vi "TEST - Empty Array.vi"(8 "error in (no error)":errorcluster) -> (0 "error out":errorcluster, 2 "Pass?":bool=TRUE)   [LabVIEW 2009]
doc: "This VI template can be used for the functional testing of VIs; this implementation includes handling for the testing of polymorphic VIs, and the polymorphic elements should be removed if not needed.\n\nCoded by Douglas A. Femec, January 24, 2006.\n\nCopyright (c) 2005-2006 MKS Instruments, Inc.\nAll rights reserved."
uses:
  TEST - Empty Array - Inputs.ctl
  Polymorphizer+ Data Type.ctl
  TEST - Empty Array - Outputs.ctl
  source/library/Empty Array/Empty 1D Array (EXT).vi
  source/library/Empty Array/Empty 2D Array (EXT).vi
  source/library/Empty Array/Empty 1D Array (I64).vi
  source/library/Empty Array/Empty 2D Array (I64).vi
  source/library/Empty Array/Empty 1D Array (U64).vi
  source/library/Empty Array/Empty 2D Array (U64).vi
  source/library/Empty Array/Empty 1D Array (DBL).vi
  source/library/Empty Array/Empty 2D Array (DBL).vi
  source/library/Empty Array/Empty 1D Array (SGL).vi
  source/library/Empty Array/Empty 2D Array (SGL).vi
  source/library/Empty Array/Empty 1D Array (I32).vi
  source/library/Empty Array/Empty 2D Array (I32).vi
  source/library/Empty Array/Empty 1D Array (I16).vi
  source/library/Empty Array/Empty 2D Array (I16).vi
  source/library/Empty Array/Empty 1D Array (I8).vi
  source/library/Empty Array/Empty 2D Array (I8).vi
  source/library/Empty Array/Empty 1D Array (LVObject).vi
  source/library/Empty Array/Empty 2D Array (LVObject).vi
  source/library/Empty Array/Empty 1D Array (U32).vi
  source/library/Empty Array/Empty 2D Array (U32).vi
  source/library/Empty Array/Empty 1D Array (U16).vi
  source/library/Empty Array/Empty 2D Array (U16).vi
  source/library/Empty Array/Empty 1D Array (U8).vi
  source/library/Empty Array/Empty 2D Array (U8).vi
  source/library/Empty Array/Empty 1D Array (CXT).vi
  source/library/Empty Array/Empty 2D Array (CXT).vi
  source/library/Empty Array/Empty 1D Array (CDB).vi
  source/library/Empty Array/Empty 2D Array (CDB).vi
  source/library/Empty Array/Empty 1D Array (CSG).vi
  source/library/Empty Array/Empty 2D Array (CSG).vi
  source/library/Empty Array/Empty 1D Array (Boolean).vi
  source/library/Empty Array/Empty 2D Array (Boolean).vi
  source/library/Empty Array/Empty 1D Array (String).vi
  source/library/Empty Array/Empty 2D Array (String).vi
  source/library/Empty Array/Empty 1D Array (Path).vi
  source/library/Empty Array/Empty 2D Array (Path).vi
  source/library/Empty Array/Empty Array (Variant).vi
  source/library/Empty Array/Empty 1D Array (Variant).vi
  source/library/Empty Array/Empty 2D Array (Variant).vi
  TestClass/TestClass.lvclass
panel:
  out "Generated Outputs":T1[][](array[typedef])
  in  "Expected Outputs":T1[](array[typedef])=[{"Description"="Expect true", "1D Empty?"=TRUE, "2D Empty?"=TRUE}, {"Description"="Expect false", "1D Empty?"=FALSE, "2D Empty?"=FALSE}, {"Description"="Expect false", "1D Empty?"=FALSE, "2D Empty?"=FALSE}]
  in  "Inputs":T2[](array[typedef])=[{"Description"="Empty arrays", "Data Types to Test"=[enum."EXT", enum."DBL", enum."SGL", enum."I32", enum."I16", enum."I8", enum."U32", enum."U16", enum."U8", enum."CXT", enum."CDB", enum."CSG", enum."Boolean", enum."String", enum."Path", enum."Variant", enum."I64", enum."U64", enum."LabVIEW Object"], "1D Array"=[], "2D Array"=[]}, {"Description"="One-element arrays", "Data Types to Test"=[enum."EXT", enum."DBL", enum."SGL", enum."I32", enum."I16", enum."I8", enum."U32", enum."U16", enum."U8", enum."CXT", enum."CDB", enum."CSG", enum."Boolean", enum."String", enum."Path", enum."Variant", enum."I64", enum."U64", enum."LabVIEW Object"], "1D Array"=[0.0], "2D Array"=[[0.0]]}, {"Description"="Multi-element arrays", "Data Types to Test"=[enum."EXT", enum."DBL", enum."SGL", enum."I32", enum."I16", enum."I8", enum."U32", enum."U16", enum."U8", enum."CXT", enum."CDB", enum."CSG", enum."Boolean", enum."String", enum."Path", enum."Variant", enum."I64", enum."U64", enum."LabVIEW Object"], "1D Array"=[1.0, 0.0, 1.0, 1.0], "2D Array"=[[0.0, 0.0], [1.0, 0.0], [1.0, 1.0]]}] {"1D Array" format="%.2f"; "2D Array" format="%.2f"}
  # "Copyright (c) 2005-2006 MKS Instruments, Inc.\nAll rights reserved."
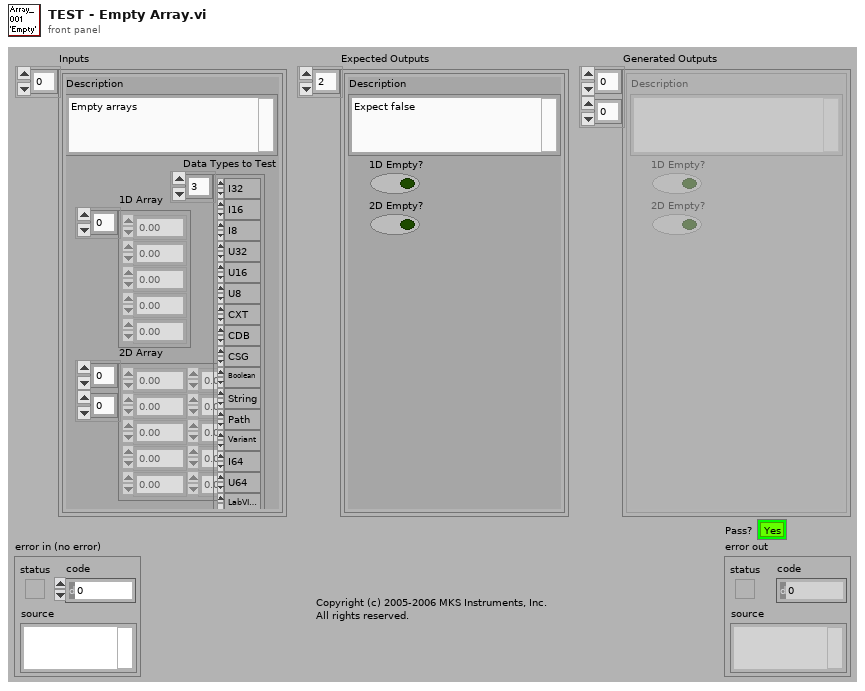
[diagram p1: front panel]
types:
  T1 = typedef "TEST - Empty Array - Outputs.ctl" = cluster{"Description":string, "1D Empty?":bool, "2D Empty?":bool}
  T2 = typedef "TEST - Empty Array - Inputs.ctl" = cluster{"Description":string, "Data Types to Test":T3[], "1D Array":sgl[], "2D Array":sgl[][]}
  T3 = typedef "Polymorphizer+ Data Type.ctl" = enum16{"EXT", "DBL", "SGL", "I32", "I16", "I8", "U32", "U16", "U8", "CXT", "CDB", "CSG", "Boolean", "String", "Path", "Variant", "CTL-REF", "GEN-REF", "GObj-REF", "VI-REF", "ENUM", "ERR", "FILE-REF", "MENU-REF", "MENU-RING", "PICT-RING", "TXT&PICT-RING", "TXT-RING", "I64", "U64", "LabVIEW Object"}
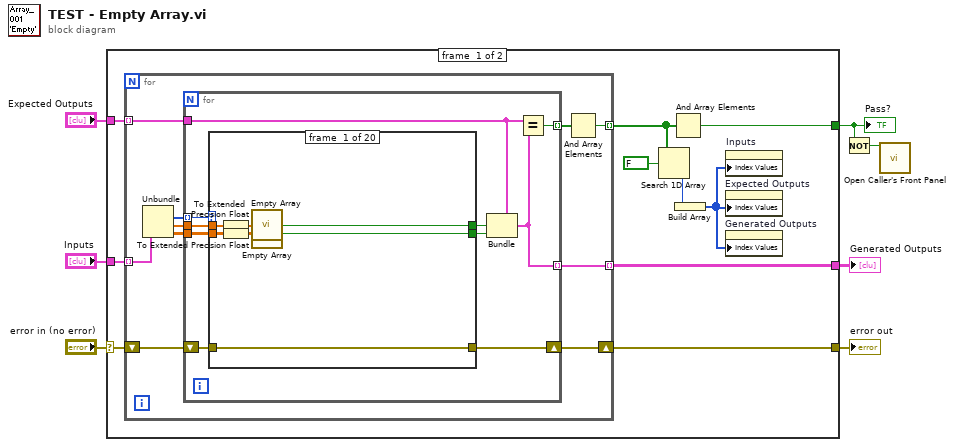
[diagram p0: block diagram]
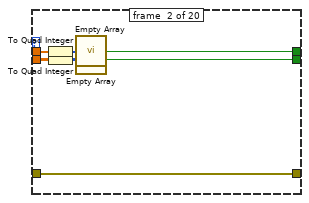
[diagram p2: hidden frame]
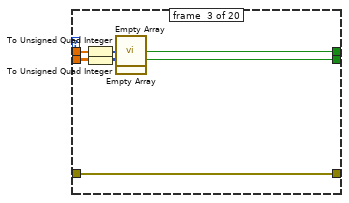
[diagram p3: hidden frame]
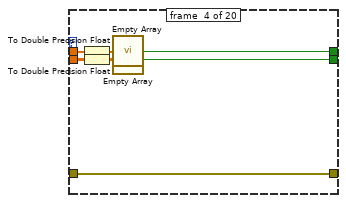
[diagram p4: hidden frame]
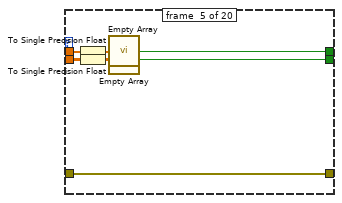
[diagram p5: hidden frame]
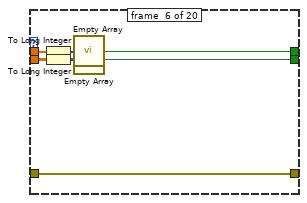
[diagram p6: hidden frame]
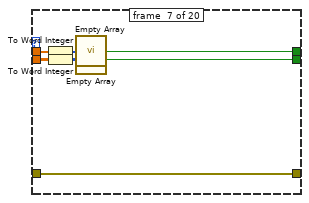
[diagram p7: hidden frame]
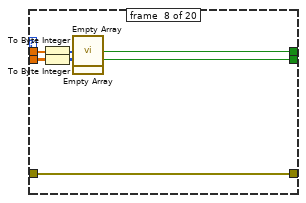
[diagram p8: hidden frame]
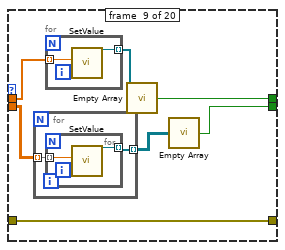
[diagram p9: hidden frame]
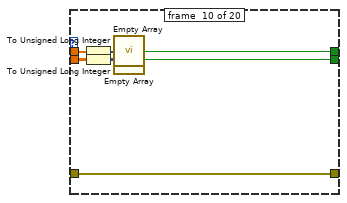
[diagram p10: hidden frame]
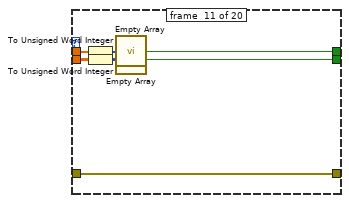
[diagram p11: hidden frame]
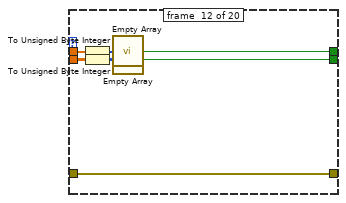
[diagram p12: hidden frame]
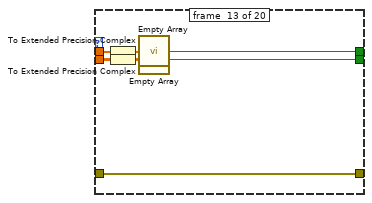
[diagram p13: hidden frame]
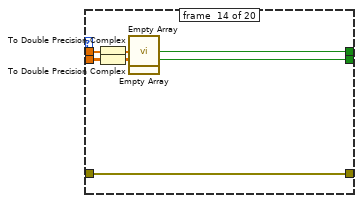
[diagram p14: hidden frame]
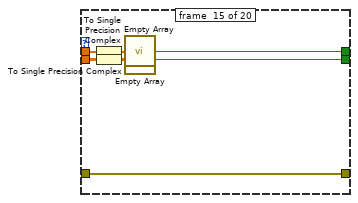
[diagram p15: hidden frame]
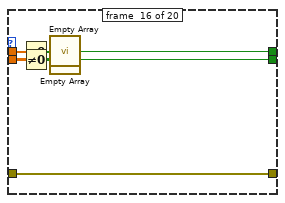
[diagram p16: hidden frame]
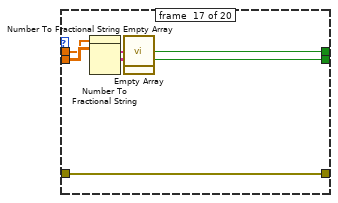
[diagram p17: hidden frame]
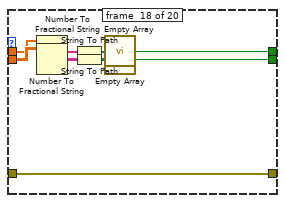
[diagram p18: hidden frame]
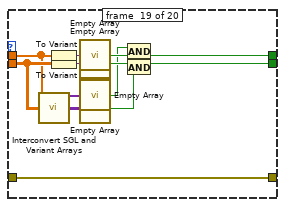
[diagram p19: hidden frame]
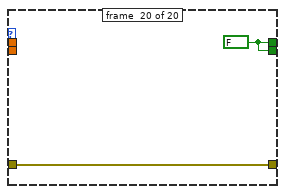
[diagram p20: hidden frame]
diagram:
  n1 = case shown="No Error" "error in (no error)" {
    selector: "error in (no error)" -> [w16 w187]
    tunnel: [w17 w187] -> w6
    tunnel: "Expected Outputs" -> [w14 _]
    tunnel: "Inputs" -> [w15 _]
    tunnel: [w13 _] -> w3
    tunnel: [w12 _] -> w1
    frame #0 {
      n2 = for {
        shift-right: [w22] -> w17
        shift-left: w16 -> [w23]
        tunnel: w15 -> [w24] mode=indexing
        tunnel: w14 -> [w27] mode=indexing
        tunnel: [w26] -> w13 mode=indexing
        tunnel: [w21] -> w11 mode=indexing
        n3 = Unbundle(w24) -> ("Data Types to Test"=w20:T3[], "1D Array"=w19:sgl[], "2D Array"=w18:sgl[][])  [unwired: 1 out]
        n4 = for {
          tunnel: w27 -> [w37]
          tunnel: [w35] -> w26 mode=indexing
          tunnel: [w36] -> w25 mode=indexing
          shift-right: [w30] -> w22
          shift-left: w23 -> [w31]
          tunnel: w20 -> [w32] mode=indexing
          tunnel: w19 -> [w34]
          tunnel: w18 -> [w33]
          n5 = case shown="\"LabVIEW Object\"" w32 {
            tunnel: w34 -> [w43 w50 w57 w64 w71 w78 w85 w92 w97 w112 w119 w126 w133 w140 w147 w154 w159 w168 w173 _]
            tunnel: [w39 w46 w53 w60 w66 w73 w80 w87 w98 w107 w114 w121 w128 w135 w142 w150 w157 w164 w177 w186] -> w29
            tunnel: [w38 w45 w52 w59 w67 w74 w81 w88 w99 w108 w115 w122 w129 w136 w143 w149 w156 w163 w175 w186] -> w28
            tunnel: w33 -> [w44 w51 w58 w65 w72 w79 w86 w93 w94 w113 w120 w127 w134 w141 w148 w155 w161 w170 w179 _]
            tunnel: w31 -> [w40 w47 w54 w61 w68 w75 w82 w89 w100 w109 w116 w123 w130 w137 w144 w151 w158 w165 w184 w185]
            tunnel: [w40 w47 w54 w61 w68 w75 w82 w89 w100 w109 w116 w123 w130 w137 w144 w151 w158 w165 w184 w185] -> w30
            frame #0 {
              n6 = To Extended Precision Float(1:w43) -> (0:w42:ext[])
              n7 = To Extended Precision Float(1:w44) -> (0:w41:ext[][])
              n8 = call-poly "Empty Array.vi"("Array"=w42) -> ("Empty Array?"=w39:bool)  [unwired: 8 in]
              n9 = call-poly "Empty Array.vi"("Array"=w41) -> ("Empty Array?"=w38:bool)  [unwired: 8 in]
            }
            frame #1 {
              n10 = To Quad Integer(1:w50) -> (0:w49:i64[])
              n11 = To Quad Integer(1:w51) -> (0:w48:i64[][])
              n12 = call-poly "Empty Array.vi"("Array"=w49) -> ("Empty Array?"=w46:bool)  [unwired: 8 in]
              n13 = call-poly "Empty Array.vi"("Array"=w48) -> ("Empty Array?"=w45:bool)  [unwired: 8 in]
            }
            frame #2 {
              n14 = To Unsigned Quad Integer(1:w57) -> (0:w56:u64[])
              n15 = To Unsigned Quad Integer(1:w58) -> (0:w55:u64[][])
              n16 = call-poly "Empty Array.vi"("Array"=w56) -> ("Empty Array?"=w53:bool)  [unwired: 8 in]
              n17 = call-poly "Empty Array.vi"("Array"=w55) -> ("Empty Array?"=w52:bool)  [unwired: 8 in]
            }
            frame #3 {
              n18 = To Double Precision Float(number=w64) -> (double precision float=w63:dbl[])
              n19 = To Double Precision Float(number=w65) -> (double precision float=w62:dbl[][])
              n20 = call-poly "Empty Array.vi"("Array"=w63) -> ("Empty Array?"=w60:bool)  [unwired: 8 in]
              n21 = call-poly "Empty Array.vi"("Array"=w62) -> ("Empty Array?"=w59:bool)  [unwired: 8 in]
            }
            frame #4 {
              n22 = To Single Precision Float(number=w71) -> (single precision float=w70:sgl[])
              n23 = To Single Precision Float(number=w72) -> (single precision float=w69:sgl[][])
              n24 = call-poly "Empty Array.vi"("Array"=w70) -> ("Empty Array?"=w66:bool)  [unwired: 8 in]
              n25 = call-poly "Empty Array.vi"("Array"=w69) -> ("Empty Array?"=w67:bool)  [unwired: 8 in]
            }
            frame #5 {
              n26 = To Long Integer(number=w78) -> (32bit integer=w77:i32[])
              n27 = To Long Integer(number=w79) -> (32bit integer=w76:i32[][])
              n28 = call-poly "Empty Array.vi"("Array"=w77) -> ("Empty Array?"=w73:bool)  [unwired: 8 in]
              n29 = call-poly "Empty Array.vi"("Array"=w76) -> ("Empty Array?"=w74:bool)  [unwired: 8 in]
            }
            frame #6 {
              n30 = To Word Integer(number=w85) -> (16bit integer=w84:i16[])
              n31 = To Word Integer(number=w86) -> (16bit integer=w83:i16[][])
              n32 = call-poly "Empty Array.vi"("Array"=w84) -> ("Empty Array?"=w80:bool)  [unwired: 8 in]
              n33 = call-poly "Empty Array.vi"("Array"=w83) -> ("Empty Array?"=w81:bool)  [unwired: 8 in]
            }
            frame #7 {
              n34 = To Byte Integer(number=w92) -> (8bit integer=w91:i8[])
              n35 = To Byte Integer(number=w93) -> (8bit integer=w90:i8[][])
              n36 = call-poly "Empty Array.vi"("Array"=w91) -> ("Empty Array?"=w87:bool)  [unwired: 8 in]
              n37 = call-poly "Empty Array.vi"("Array"=w90) -> ("Empty Array?"=w88:bool)  [unwired: 8 in]
            }
            frame #8 {
              n38 = for {
                tunnel: w94 -> [w102] mode=indexing
                tunnel: [w101] -> w95 mode=indexing
                n39 = for {
                  tunnel: w102 -> [w104] mode=indexing
                  tunnel: [w103] -> w101 mode=indexing
                  n40 = call "SetValue.vi"("Value"=w104) -> ("TestClass out"=w103:refnum<class "TestClass.lvclass">)  [unwired: 9 in, 1 out]
                }
              }
              n41 = for {
                tunnel: w97 -> [w106] mode=indexing
                tunnel: [w105] -> w96 mode=indexing
                n42 = call "SetValue.vi"("Value"=w106) -> ("TestClass out"=w105:refnum<class "TestClass.lvclass">)  [unwired: 9 in, 1 out]
              }
              n43 = call-poly "Empty Array.vi"("Array"=w96) -> ("Empty Array?"=w98:bool)  [unwired: 8 in]
              n44 = call-poly "Empty Array.vi"("Array"=w95) -> ("Empty Array?"=w99:bool)  [unwired: 8 in]
            }
            frame #9 {
              n45 = To Unsigned Long Integer(number=w112) -> (unsigned 32bit integer=w111:u32[])
              n46 = To Unsigned Long Integer(number=w113) -> (unsigned 32bit integer=w110:u32[][])
              n47 = call-poly "Empty Array.vi"("Array"=w111) -> ("Empty Array?"=w107:bool)  [unwired: 8 in]
              n48 = call-poly "Empty Array.vi"("Array"=w110) -> ("Empty Array?"=w108:bool)  [unwired: 8 in]
            }
            frame #10 {
              n49 = To Unsigned Word Integer(number=w119) -> (unsigned 16bit integer=w118:u16[])
              n50 = To Unsigned Word Integer(number=w120) -> (unsigned 16bit integer=w117:u16[][])
              n51 = call-poly "Empty Array.vi"("Array"=w118) -> ("Empty Array?"=w114:bool)  [unwired: 8 in]
              n52 = call-poly "Empty Array.vi"("Array"=w117) -> ("Empty Array?"=w115:bool)  [unwired: 8 in]
            }
            frame #11 {
              n53 = To Unsigned Byte Integer(number=w126) -> (unsigned 8bit integer=w125:u8[])
              n54 = To Unsigned Byte Integer(number=w127) -> (unsigned 8bit integer=w124:u8[][])
              n55 = call-poly "Empty Array.vi"("Array"=w125) -> ("Empty Array?"=w121:bool)  [unwired: 8 in]
              n56 = call-poly "Empty Array.vi"("Array"=w124) -> ("Empty Array?"=w122:bool)  [unwired: 8 in]
            }
            frame #12 {
              n57 = To Extended Precision Complex(1:w133) -> (0:w132:cxt[])
              n58 = To Extended Precision Complex(1:w134) -> (0:w131:cxt[][])
              n59 = call-poly "Empty Array.vi"("Array"=w132) -> ("Empty Array?"=w128:bool)  [unwired: 8 in]
              n60 = call-poly "Empty Array.vi"("Array"=w131) -> ("Empty Array?"=w129:bool)  [unwired: 8 in]
            }
            frame #13 {
              n61 = To Double Precision Complex(1:w140) -> (0:w139:cdb[])
              n62 = To Double Precision Complex(1:w141) -> (0:w138:cdb[][])
              n63 = call-poly "Empty Array.vi"("Array"=w139) -> ("Empty Array?"=w135:bool)  [unwired: 8 in]
              n64 = call-poly "Empty Array.vi"("Array"=w138) -> ("Empty Array?"=w136:bool)  [unwired: 8 in]
            }
            frame #14 {
              n65 = To Single Precision Complex(1:w147) -> (0:w146:csg[])
              n66 = To Single Precision Complex(1:w148) -> (0:w145:csg[][])
              n67 = call-poly "Empty Array.vi"("Array"=w146) -> ("Empty Array?"=w142:bool)  [unwired: 8 in]
              n68 = call-poly "Empty Array.vi"("Array"=w145) -> ("Empty Array?"=w143:bool)  [unwired: 8 in]
            }
            frame #15 {
              n69 = Not Equal To 0?(x=w154) -> (x != 0?=w153:bool[])
              n70 = Not Equal To 0?(x=w155) -> (x != 0?=w152:bool[][])
              n71 = call-poly "Empty Array.vi"("Array"=w153) -> ("Empty Array?"=w150:bool)  [unwired: 8 in]
              n72 = call-poly "Empty Array.vi"("Array"=w152) -> ("Empty Array?"=w149:bool)  [unwired: 8 in]
            }
            frame #16 {
              n73 = Number To Fractional String(number=w159) -> (F-format string=w160:string[])  [unwired: 3 in]
              n74 = Number To Fractional String(number=w161) -> (F-format string=w162:string[][])  [unwired: 3 in]
              n75 = call-poly "Empty Array.vi"("Array"=w160) -> ("Empty Array?"=w157:bool)  [unwired: 8 in]
              n76 = call-poly "Empty Array.vi"("Array"=w162) -> ("Empty Array?"=w156:bool)  [unwired: 8 in]
            }
            frame #17 {
              n77 = Number To Fractional String(number=w168) -> (F-format string=w169:string[])  [unwired: 3 in]
              n78 = Number To Fractional String(number=w170) -> (F-format string=w171:string[][])  [unwired: 3 in]
              n79 = String To Path(string=w169) -> (path=w166:path[])
              n80 = String To Path(string=w171) -> (path=w167:path[][])
              n81 = call-poly "Empty Array.vi"("Array"=w166) -> ("Empty Array?"=w164:bool)  [unwired: 8 in]
              n82 = call-poly "Empty Array.vi"("Array"=w167) -> ("Empty Array?"=w163:bool)  [unwired: 8 in]
            }
            frame #18 {
              n83 = call "Interconvert SGL and Variant Arrays.vi"("SGL 1D Array In"=w173, "SGL 2D Array In"=w179) -> ("Variant 1D Array Out"=w172:variant[], "Variant 2D Array Out"=w178:variant[][])  [unwired: 9 in, 3 out]
              n84 = To Variant(anything=w173) -> (Variant=w182:variant)
              n85 = To Variant(anything=w179) -> (Variant=w183:variant)
              n86 = call-poly "Empty Array.vi"("Array"=w182) -> ("Empty Array?"=w181:bool)  [unwired: 8 in]
              n87 = call-poly "Empty Array.vi"("Array"=w183) -> ("Empty Array?"=w180:bool)  [unwired: 8 in]
              n88 = call-poly "Empty Array.vi"("Array"=w172) -> ("Empty Array?"=w176:bool)  [unwired: 8 in]
              n89 = call-poly "Empty Array.vi"("Array"=w178) -> ("Empty Array?"=w174:bool)  [unwired: 8 in]
              n90 = And(x=w176, y=w181) -> (x .and. y?=w177:bool)
              n91 = And(x=w180, y=w174) -> (x .and. y?=w175:bool)
            }
            frame #19 {
              w186 = FALSE ("Empty Array?")
            }
          }
          n92 = Bundle(cluster=w37, "1D Empty?"=w29, "2D Empty?"=w28) -> (w35:T1)  [unwired: 1 in]
          n93 = Equal?(x=w37, y=w35) -> (x = y?=w36:bool)
        }
        n94 = And Array Elements(Boolean array=w25) -> (logical AND=w21:bool)
      }
      n95 = Search 1D Array(1D array=w11, element=FALSE) -> (index of element=w9:i32)  [unwired: 1 in]
      n96 = And Array Elements(Boolean array=w11) -> (logical AND=w12:bool)
      n97 = Build Array(w9) -> (w8:i32[])
      n98 = property on="Inputs" class="Arr (strict)"("Index Values"=w8) -> ()  [unwired: 2 in, 2 out]
      n99 = property on="Expected Outputs" class="Arr (strict)"("Index Values"=w8) -> ()  [unwired: 2 in, 2 out]
      n100 = property on="Generated Outputs" class="Arr (strict)"("Index Values"=w8) -> ()  [unwired: 2 in, 2 out]
    }
    frame #1 {
    }
  }
  "error out" <- w6
  "Pass?" <- w1
  "Generated Outputs" <- w3
  n101 = Not(x=w1) -> (.not. x?=w2:bool)
  n102 = call "Open Caller's Front Panel.vi"("Open?"=w2) -> ()  [unwired: 14 in, 1 out]
